vi "Main.vi"() -> ()   [LabVIEW 2017, in "My Singleton Module.lvlib"]
doc: "This template is based from the Queued Message Handler design pattern and the Queued Message Handler Project Template that ships with LabVIEW 2014.\n\nThe main difference is that the Queue is private to this module and communication between modules is done via Broadcast and Request events.\n\nRequest events are wrapped via public API methods and are handled in the Event handler loop in this VI.\nAny module can register for Broadcast events sent by this module.\n\nThe Event Handling Loop generates messages based on user interface actions.\n\nThe Message Handling Loop processes messages generated by the Event Handling Loop, or by other messages. The messages are string values, so new messages can be added easily to the Message Cases case structure in the Message Handling Loop. Each message cluster can also provide an optional value for Message Data, which is a variant that can be converted to whatever message-specific data is required.\n_____\nBased on Delacor QMH Project Template 3.1.0.34."
uses:
  My Singleton Module.lvlib
  <vilib>/Delacor/Delacor QMH/Libraries/Module Admin_class/Delacor_lib_QMH_Module Admin.lvclass
  Module Data--cluster.ctl
  Do Something Else Argument--cluster.ctl
  Do Something Else and Wait for Reply Argument--cluster.ctl
  Do Something Else and Wait (Reply Payload)--cluster.ctl
  Show Panel Argument--cluster.ctl
  Hide Panel Argument--cluster.ctl
  Stop Argument--cluster.ctl
  <vilib>/Delacor/Delacor QMH/Libraries/Module Admin_class/Delacor_lib_QMH_Module Admin.lvclass/Delacor_lib_QMH_Module Admin.ctl
  <vilib>/Utility/miscctls.llb/LVPointTypeDef.ctl
  <vilib>/Delacor/Delacor QMH/Libraries/Module Admin_class/Delacor_lib_QMH_Get External Launch.vi
  <vilib>/Delacor/Delacor QMH/Libraries/Message Queue_class/Delacor_lib_QMH_Enqueue Message (Single).vi
  <vilib>/Utility/error.llb/Error Cluster From Error Code.vi
  <vilib>/ErrorRing/Error Ring.xnode
  <vilib>/Delacor/Delacor QMH/Libraries/Message Queue_class/Delacor_lib_QMH_Message Queue.lvclass
panel:
  in  "Simulate MHL Error":bool
  in  "Simulate EHL Error":bool
  out "error out":errorcluster
  in  "Module Admin":refnum<class "Delacor_lib_QMH_Module Admin.lvclass">
  out "X":dbl
  out "Status":string
  in  "Do Something Else <Replace Me>":bool
  in  "Do Something <Replace Me>":bool
  # "These controls have associated \"Value Changed\" events configured in the Event Structure on the diagram.\n\nReplace them (and reconfigure the Event Structure) with the controls you need for your application. \n\nOther QMH Modules communicate with this Module via its Public API (wrappers for its Request Events).\n\nThis Module communicates with other Modules via its Broadcast Events.\nAny module that wants to get these messages, just registers for this module's Broadcast events."
  # "This template is for the Delacor Modified Queued Message Handler design pattern.\n\nSee the block diagram for more information on how to use this template."
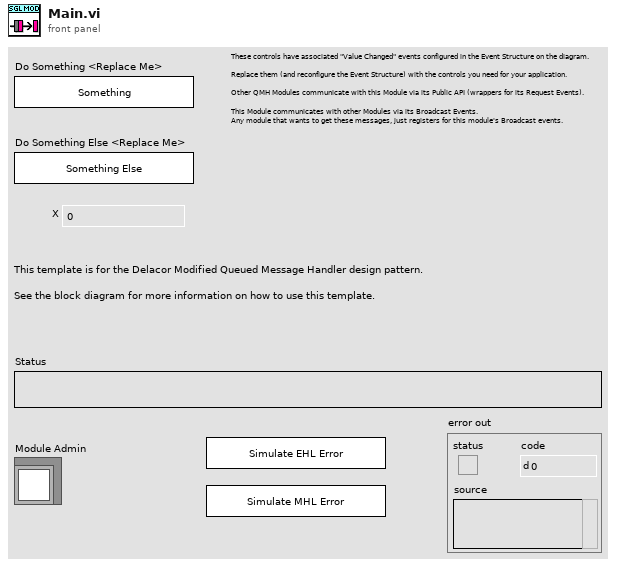
[diagram p1: front panel]
types:
  T1 = typedef "My Singleton Module.lvlib/Request Events--cluster.ctl" = cluster{"Stop Module":refnum<user-event>, "Do Something":refnum<user-event>, "Do Something Else":refnum<user-event>, "Do Something Else and Wait for Reply":refnum<user-event>, "Show Panel":refnum<user-event>, "Hide Panel":refnum<user-event>, "Get Module Execution Status":refnum<user-event>, "Show Diagram":refnum<user-event>}
  T2 = typedef "My Singleton Module.lvlib/Module Data--cluster.ctl" = cluster{"Status":string}
  T3 = typedef "My Singleton Module.lvlib/Do Something Else Argument--cluster.ctl" = cluster{"Do Something Else Msg":string, "X":dbl}
  T4 = typedef "My Singleton Module.lvlib/Do Something Else and Wait for Reply Argument--cluster.ctl" = cluster{"Do Something Else Msg":string, "X":dbl, "Wait Notifier":refnum<notifier>}
  T5 = typedef "My Singleton Module.lvlib/Show Panel Argument--cluster.ctl" = cluster{"Show Panel?":bool}
  T6 = typedef "My Singleton Module.lvlib/Hide Panel Argument--cluster.ctl" = cluster{"Hide Panel?":bool}
  T7 = typedef "My Singleton Module.lvlib/Stop Argument--cluster.ctl" = cluster{"Origin":string, "Exit via Stop Module Req?":bool, "Wait for Module to stop?":bool}
  T8 = typedef "LVPointTypeDef.ctl" = cluster{"Horizontal":i16, "Vertical":i16}
  T9 = enum32{"Invalid", "Standard", "Closed", "Hidden", "Minimized", "Maximized"}
  T10 = enum32{"invalid lock state", "Not Locked", "Locked (No Password)", "Password-protected"}
  T11 = typedef "My Singleton Module.lvlib/Do Something Else and Wait (Reply Payload)--cluster.ctl" = cluster{"Value":dbl, "error":errorcluster}
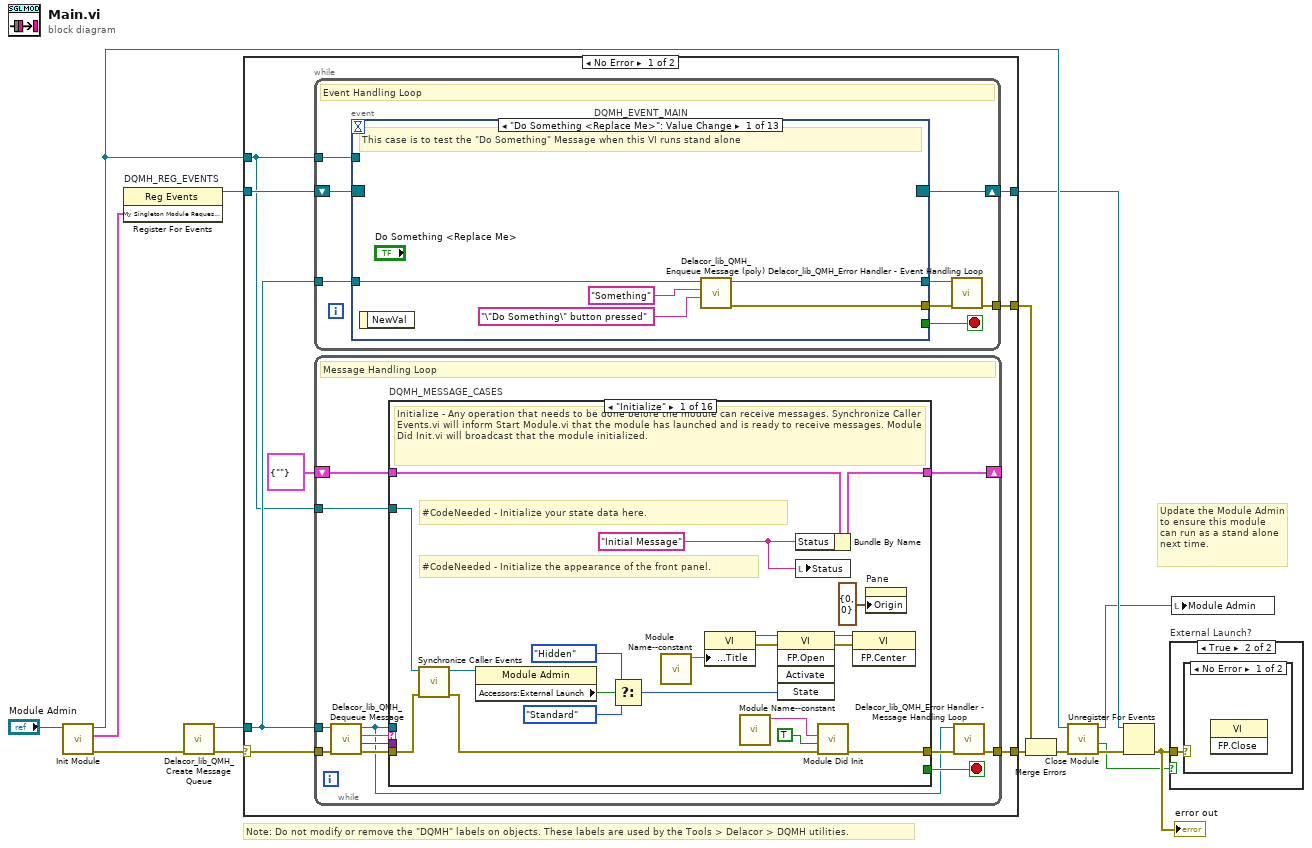
[diagram p0: block diagram]
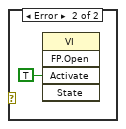
[diagram p3: hidden frame]
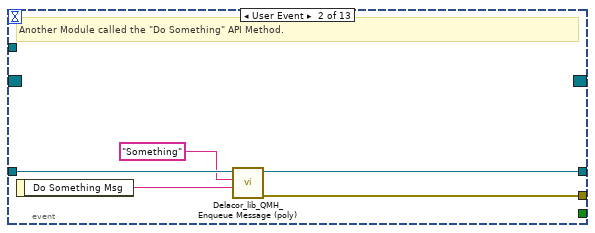
[diagram p4: hidden frame]
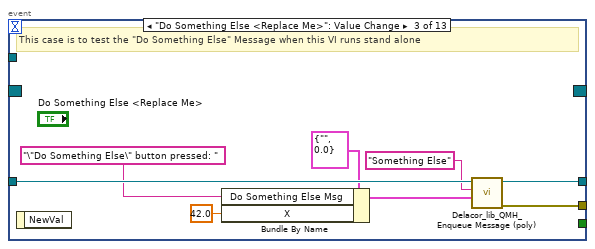
[diagram p5: hidden frame]
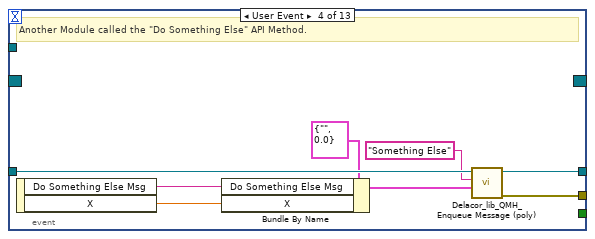
[diagram p6: hidden frame]
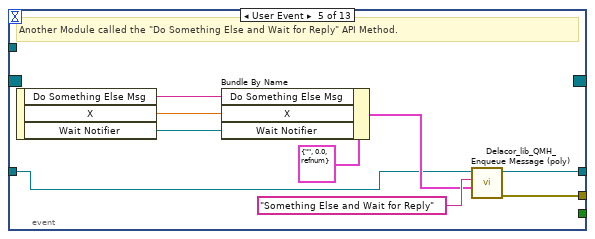
[diagram p7: hidden frame]
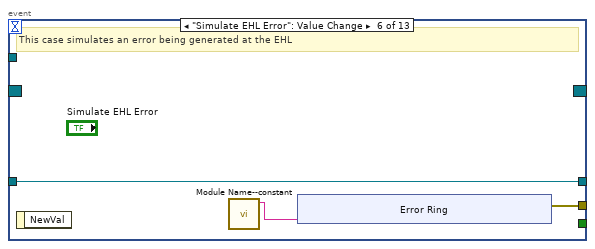
[diagram p8: hidden frame]
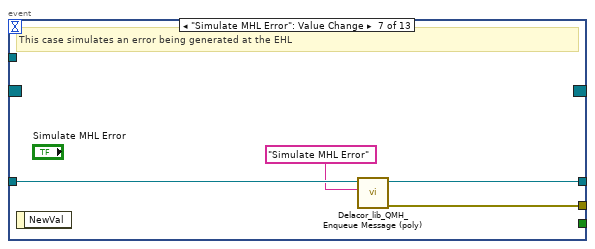
[diagram p9: hidden frame]
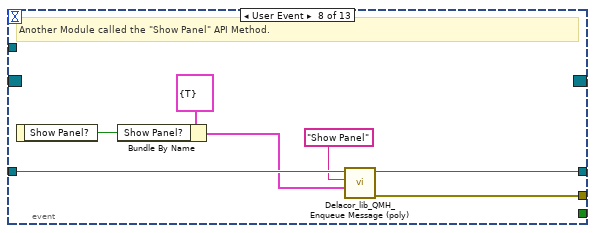
[diagram p10: hidden frame]
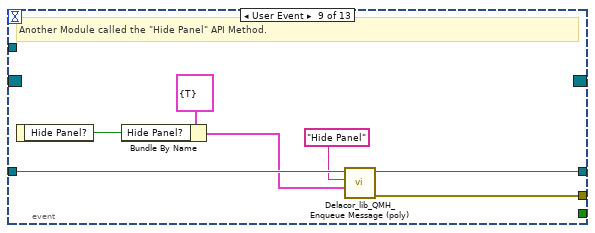
[diagram p11: hidden frame]
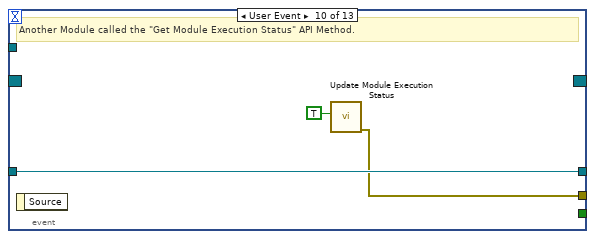
[diagram p12: hidden frame]
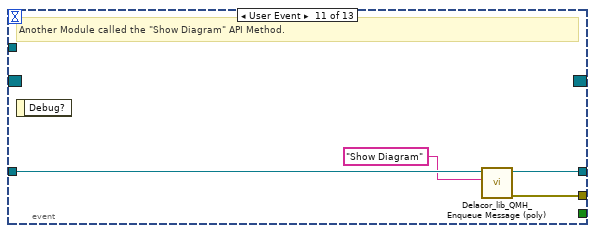
[diagram p13: hidden frame]
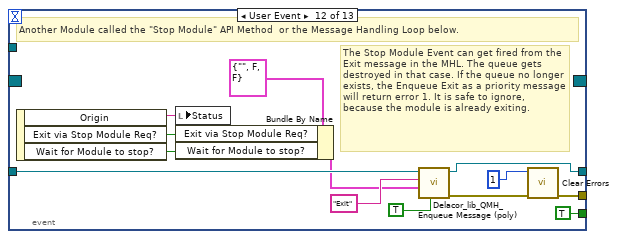
[diagram p14: hidden frame]
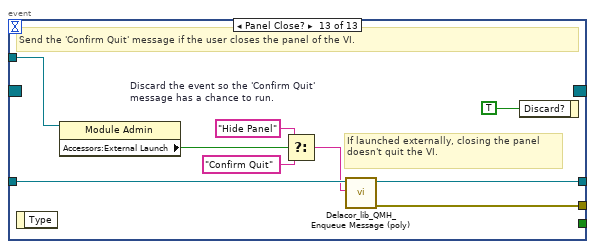
[diagram p15: hidden frame]
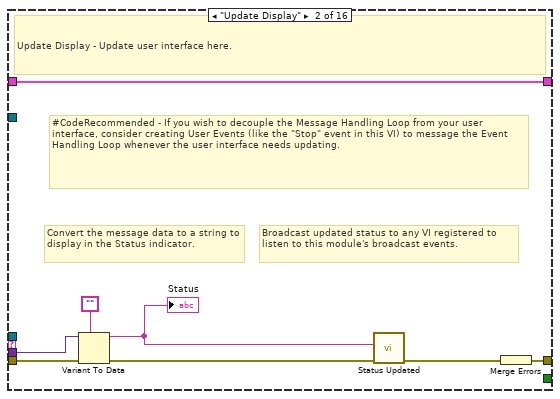
[diagram p16: hidden frame]
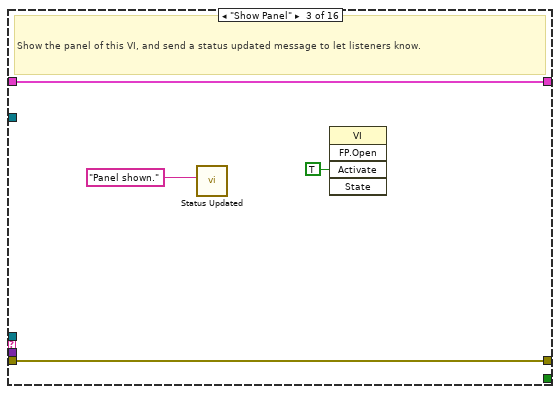
[diagram p17: hidden frame]
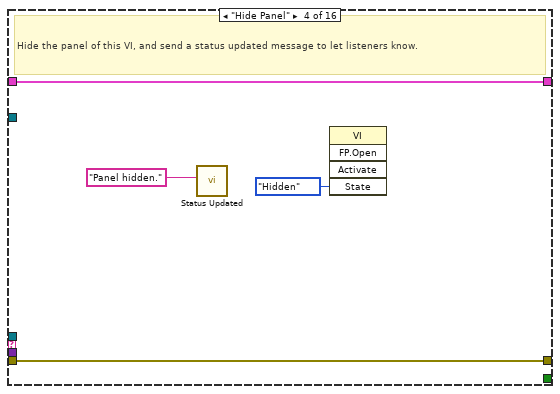
[diagram p18: hidden frame]
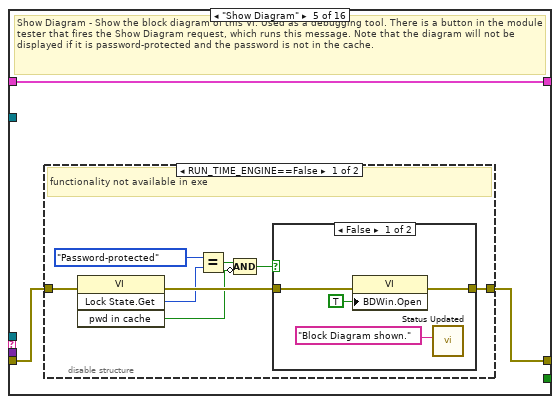
[diagram p19: hidden frame]
diagram:
  # "Note: Do not modify or remove the \"DQMH\" labels on objects. These labels are used by the Tools > Delacor > DQMH utilities."
  # "Update the Module Admin to ensure this module can run as a stand alone next time."
  n1 = call "Init Module.vi"("Singleton Module Admin in"="Module Admin") -> ("error out"=w13:errorcluster, "My Singleton Module Request Events"=w10:T1, "Singleton Module Admin out"=w15:refnum<class "Delacor_lib_QMH_Module Admin.lvclass">)  [unwired: 8 in]
  n2 = register-events "DQMH_REG_EVENTS"(w10) -> (reference out=w11:refnum<event-registration>)  [unwired: 2 in, 1 out]
  n3 = call <vilib>:"Delacor_lib_QMH_Create Message Queue.vi"("error in (no error)"=w13) -> ("error out"=w1:errorcluster, "Message Queue out"=w9:refnum<class "Delacor_lib_QMH_Message Queue.lvclass">)  [unwired: 9 in]
  n4 = case shown="No Error" w1 {
    selector: w1 -> [w17 w316]
    tunnel: [w23 w316] -> w14
    tunnel: [w22 w321] -> w12
    tunnel: w11 -> [w20 w321]
    tunnel: w9 -> [w19 _]
    tunnel: [w18 _] -> w5
    tunnel: w15 -> [w16 w317]
    frame No Error {
      n5 = while {
        tunnel: w19 -> [w31]
        shift-right: [w29] -> w22
        shift-left: w20 -> [w30]
        tunnel: [w25] -> w18
        tunnel: w16 -> [w24]
        stop <- w27 stop-if-true
        # "Event Handling Loop"
        n6 = event "DQMH_EVENT_MAIN" shown="[0] \"Do Something <Replace Me>\": Value Change" {
          selector: w30 -> [_ _ _ _ _ _ _ _ _ _ _ _ _]
          dyn-events: [_ _ _ _ _ _ _ _ _ _ _ _ _] -> w29
          timeout: _ -> [_ _ _ _ _ _ _ _ _ _ _ _ _]
          tunnel: [_ _ _ _ _ _ _ _ _ _ _ TRUE ("Discard?") _] -> w27
          tunnel: w31 -> [w36 w41 w49 w57 w58 w69 w80 w87 w94 w97 w101 w112 w122]
          tunnel: [w33 w38 w46 w54 w64 w68 w77 w85 w92 w96 w98 w106 w121] -> w28
          tunnel: [w35 w40 w48 w56 w66 w69 w79 w86 w93 w97 w100 w111 w120] -> w26
          tunnel: w24 -> [_ _ _ _ _ _ _ _ _ _ _ _ w116]
          event "Do Something <Replace Me>": Value Change {
            # "This case is to test the \"Do Something\" Message when this VI runs stand alone"
            n7 = event-data() -> ()  [unwired: 1 in, 1 out]
            n8 = call-poly <vilib>:"Delacor_lib_QMH_Enqueue Message (poly).vi"("Message Data"="\"Do Something\" button pressed" ("\"Do Something\" button pressed"), "Message"="Something", "Message Queue in"=w36) -> ("error out"=w33:errorcluster, "Message Queue out"=w35:refnum<class "Delacor_lib_QMH_Message Queue.lvclass">)  [unwired: 7 in]
          }
          event User Event {
            # "Another Module called the \"Do Something\" API Method."
            n9 = event-data() -> ("Do Something Msg"=w37:string)  [unwired: 1 in]
            n10 = call-poly <vilib>:"Delacor_lib_QMH_Enqueue Message (poly).vi"("Message Data"=w37, "Message"="Something", "Message Queue in"=w41) -> ("error out"=w38:errorcluster, "Message Queue out"=w40:refnum<class "Delacor_lib_QMH_Message Queue.lvclass">)  [unwired: 7 in]
          }
          event "Do Something Else <Replace Me>": Value Change {
            # "This case is to test the \"Do Something Else\" Message when this VI runs stand alone"
            n11 = event-data() -> ()  [unwired: 1 in, 1 out]
            n12 = Bundle By Name(cluster=T3 {"Do Something Else Msg"="", "X"=0.0} ("Do Something Else Argument"), "Do Something Else Msg"="\"Do Something Else\" button pressed: " ("\"Do Something Else\" button pressed"), "X"=42.0) -> (w44:T3)
            n13 = call-poly <vilib>:"Delacor_lib_QMH_Enqueue Message (poly).vi"("Message Data"=w44, "Message"="Something Else", "Message Queue in"=w49) -> ("error out"=w46:errorcluster, "Message Queue out"=w48:refnum<class "Delacor_lib_QMH_Message Queue.lvclass">)  [unwired: 7 in]
          }
          event User Event {
            # "Another Module called the \"Do Something Else\" API Method."
            n14 = event-data() -> ("Do Something Else Msg"=w51:string, "X"=w50:dbl)  [unwired: 1 in]
            n15 = Bundle By Name(cluster=T3 {"Do Something Else Msg"="", "X"=0.0} ("Do Something Else Argument"), "Do Something Else Msg"=w51, "X"=w50) -> (w52:T3)
            n16 = call-poly <vilib>:"Delacor_lib_QMH_Enqueue Message (poly).vi"("Message Data"=w52, "Message"="Something Else", "Message Queue in"=w57) -> ("error out"=w54:errorcluster, "Message Queue out"=w56:refnum<class "Delacor_lib_QMH_Message Queue.lvclass">)  [unwired: 7 in]
          }
          event User Event {
            # "Another Module called the \"Do Something Else and Wait for Reply\" API Method."
            n17 = event-data() -> ("Do Something Else Msg"=w61:string, "X"=w60:dbl, "Wait Notifier"=w59:refnum<notifier>)  [unwired: 1 in]
            n18 = Bundle By Name(cluster=T4 {"Do Something Else Msg"="", "X"=0.0, "Wait Notifier"=refnum} ("Do Something Else and Wait for Reply Argument"), "Do Something Else Msg"=w61, "X"=w60, "Wait Notifier"=w59) -> (w62:T4)
            n19 = call-poly <vilib>:"Delacor_lib_QMH_Enqueue Message (poly).vi"("Message Data"=w62, "Message"="Something Else and Wait for Reply", "Message Queue in"=w58) -> ("error out"=w64:errorcluster, "Message Queue out"=w66:refnum<class "Delacor_lib_QMH_Message Queue.lvclass">)  [unwired: 7 in]
          }
          event "Simulate EHL Error": Value Change {
            # "This case simulates an error being generated at the EHL"
            n20 = event-data() -> ()  [unwired: 1 in, 1 out]
            n21 = call "Module Name--constant.vi"() -> ("Module Name"=w67:string)  [unwired: 11 in]
            n22 = xnode "Error Ring"("parameter 0"=w67) -> ("error out"=w68:errorcluster)
          }
          event "Simulate MHL Error": Value Change {
            # "This case simulates an error being generated at the EHL"
            n23 = event-data() -> ()  [unwired: 1 in, 1 out]
            n24 = call-poly <vilib>:"Delacor_lib_QMH_Enqueue Message (poly).vi"("Message"="Simulate MHL Error", "Message Queue in"=w80) -> ("error out"=w77:errorcluster, "Message Queue out"=w79:refnum<class "Delacor_lib_QMH_Message Queue.lvclass">)  [unwired: 8 in]
          }
          event User Event {
            # "Another Module called the \"Show Panel\" API Method."
            n25 = event-data() -> ("Show Panel?"=w83:bool)  [unwired: 1 in]
            n26 = Bundle By Name(cluster=T5 {"Show Panel?"=TRUE} ("Show Panel Argument"), "Show Panel?"=w83) -> (w81:T5)
            n27 = call-poly <vilib>:"Delacor_lib_QMH_Enqueue Message (poly).vi"("Message Data"=w81, "Message"="Show Panel", "Message Queue in"=w87) -> ("error out"=w85:errorcluster, "Message Queue out"=w86:refnum<class "Delacor_lib_QMH_Message Queue.lvclass">)  [unwired: 7 in]
          }
          event User Event {
            # "Another Module called the \"Hide Panel\" API Method."
            n28 = event-data() -> ("Hide Panel?"=w89:bool)  [unwired: 1 in]
            n29 = Bundle By Name(cluster=T6 {"Hide Panel?"=TRUE} ("Hide Panel Argument"), "Hide Panel?"=w89) -> (w88:T6)
            n30 = call-poly <vilib>:"Delacor_lib_QMH_Enqueue Message (poly).vi"("Message Data"=w88, "Message"="Hide Panel", "Message Queue in"=w94) -> ("error out"=w92:errorcluster, "Message Queue out"=w93:refnum<class "Delacor_lib_QMH_Message Queue.lvclass">)  [unwired: 7 in]
          }
          event User Event {
            # "Another Module called the \"Get Module Execution Status\" API Method."
            n31 = event-data() -> ()  [unwired: 1 in, 1 out]
            n32 = call "Update Module Execution Status.vi"("Running?"=TRUE) -> ("error out"=w96:errorcluster)  [unwired: 10 in]
          }
          event User Event {
            # "Another Module called the \"Show Diagram\" API Method."
            n33 = event-data() -> ()  [unwired: 1 in, 1 out]
            n34 = call-poly <vilib>:"Delacor_lib_QMH_Enqueue Message (poly).vi"("Message"="Show Diagram", "Message Queue in"=w101) -> ("error out"=w98:errorcluster, "Message Queue out"=w100:refnum<class "Delacor_lib_QMH_Message Queue.lvclass">)  [unwired: 8 in]
          }
          event User Event {
            # "The Stop Module Event can get fired from the Exit message in the MHL. The queue gets destroyed in that case. If the queue no longer exists, the Enqueue Exit as a priority message will return error 1. It is safe to ignore, because the module is already exiting."
            # "Another Module called the \"Stop Module\" API Method  or the Message Handling Loop below."
            n35 = event-data() -> ("Origin"=w110:string, "Exit via Stop Module Req?"=w104:bool, "Wait for Module to stop?"=w103:bool)  [unwired: 1 in]
            n36 = local write "Status"(w110) -> ()
            n37 = Bundle By Name(cluster=T7 {"Origin"="", "Exit via Stop Module Req?"=FALSE, "Wait for Module to stop?"=FALSE} ("Stop Argument"), "Exit via Stop Module Req?"=w104, "Wait for Module to stop?"=w103) -> (w102:T7)
            n38 = call-poly <vilib>:"Delacor_lib_QMH_Enqueue Message (poly).vi"("Priority Message? (F)"=TRUE, "Message Data"=w102, "Message"="Exit", "Message Queue in"=w112) -> ("error out"=w107:errorcluster, "Message Queue out"=w111:refnum<class "Delacor_lib_QMH_Message Queue.lvclass">)  [unwired: 6 in]
            n39 = call <vilib>:"Clear Errors.vi"("error in (no error)"=w107, "specific error code to clear (0: all)"=1) -> ("error out"=w106:errorcluster)  [unwired: 4 in, 1 out]
          }
          event Panel Close? {
            w123 = TRUE  # Discard the event so the 'Confirm Quit' message has a chance to run.
            # "If launched externally, closing the panel doesn't quit the VI."
            # "Send the 'Confirm Quit' message if the user closes the panel of the VI."
            n40 = event-data() -> ()  [unwired: 1 in, 1 out]
            n41 = property class="Module Admin"(reference=w116) -> ("Accessors:External Launch"=w115:bool)  [unwired: 1 in, 2 out]
            n42 = Select(t="Hide Panel" ("Message"), s=w115, f="Confirm Quit" ("Message")) -> (s? t:f=w117:string)
            n43 = call-poly <vilib>:"Delacor_lib_QMH_Enqueue Message (poly).vi"("Message"=w117, "Message Queue in"=w122) -> ("error out"=w121:errorcluster, "Message Queue out"=w120:refnum<class "Delacor_lib_QMH_Message Queue.lvclass">)  [unwired: 8 in]
            n44 = event-data("Discard?"=w123) -> ()  [unwired: 1 in, 1 out]
          }
        }
        n45 = call-dynamic "Delacor_lib_QMH_Error Handler - Event Handling Loop.vi"("error in (no error)"=w28, "Message Queue in"=w26) -> ("dup error in"=w25:errorcluster)  [unwired: 8 in, 1 out]
      }
      n46 = while {
        tunnel: w19 -> [w127]
        shift-right: [w133] -> _
        shift-left: T2 {"Status"=""} ("Data Cluster") -> [w134]
        tunnel: w17 -> [w131]
        tunnel: [w125] -> w23
        tunnel: w16 -> [w124]
        stop <- w132 stop-if-true
        # "Message Handling Loop"
        n47 = call-dynamic "Delacor_lib_QMH_Dequeue Message.vi"("error in (no error)"=w131, "Message Queue in"=w127) -> ("error out"=w130:errorcluster, "Message Data"=w128:variant, "Message"=w129:string, "Message Queue out"=w126:refnum<class "Delacor_lib_QMH_Message Queue.lvclass">)  [unwired: 6 in]
        n48 = case "DQMH_MESSAGE_CASES" shown="\"Initialize\"" w129 {
          selector: w129 -> [_ _ _ _ _ _ _ _ _ _ _ _ _ _ _ w303]
          tunnel: w126 -> [_ _ _ _ _ _ w197 w212 w235 _ _ _ w267 w282 w299 _]
          tunnel: w130 -> [w145 w161 w167 w168 w173 w191 w202 w210 w233 w248 w251 w256 w273 w286 w301 _]
          tunnel: [w138 w162 w167 w168 w172 w189 w199 w214 w217 w246 w249 w254 w264 w284 w295 w304] -> w135
          tunnel: w134 -> [w144 w163 w166 w171 w174 w190 w200 w215 w237 w247 w250 w255 w272 w285 w298 w305]
          tunnel: [w143 w163 w166 w171 w174 w190 w200 w215 w237 w247 w250 w255 w272 w285 w298 w305] -> w133
          tunnel: [_ _ _ _ _ _ _ _ _ _ _ _ _ _ w297 _] -> w132
          tunnel: w128 -> [_ w160 _ _ _ _ w194 w206 w229 _ _ _ w271 _ w294 _]
          tunnel: w124 -> [w146 _ _ _ _ _ _ _ _ _ _ _ w266 _ w287 _]
          frame "Initialize" {
            w142 = "Initial Message" ("Initial Message")
            # "#CodeNeeded - Initialize the appearance of the front panel."
            # "#CodeNeeded - Initialize your state data here."
            # "Initialize - Any operation that needs to be done before the module can receive messages. Synchronize Caller Events.vi will inform Start Module.vi that the module has launched and is ready to receive messages. Module Did Init.vi will broadcast that the module initialized."
            n49 = call "Synchronize Caller Events.vi"("error in (no error)"=w145, "Singleton Module Admin in"=w146) -> ("error out"=w139:errorcluster, "Singleton Module Admin out"=w137:refnum<class "Delacor_lib_QMH_Module Admin.lvclass">)  [unwired: 8 in]
            n50 = property class="Module Admin"(reference=w137) -> ("Accessors:External Launch"=w150:bool)  [unwired: 1 in, 2 out]
            n51 = Select(t=T9."Hidden" ("State"), s=w150, f=T9."Standard" ("State")) -> (s? t:f=w147:T9)
            n52 = call "Module Name--constant.vi"() -> ("Module Name"=w155:string)  [unwired: 11 in]
            n53 = property class="VI"("Front Panel.Title"=w155) -> (reference out=w153:refnum<vi>, error out=w154:errorcluster)  [unwired: 2 in]
            n54 = call "Module Name--constant.vi"() -> ("Module Name"=w140:string)  [unwired: 11 in]
            n55 = invoke class="VI" method="FP.Open"(reference=w153, error in=w154, "State"=w147) -> (reference out=w152:refnum<vi>, error out=w151:errorcluster)  [unwired: 2 in, 3 out]
            n56 = Bundle By Name(cluster=w144, "Status"=w142) -> (w143:T2)
            n57 = local write "Status"(w142) -> ()
            n58 = call "Module Did Init.vi"("error in (no error)"=w139, "Initialized?"=TRUE, "Origin"=w140) -> ("error out"=w138:errorcluster)  [unwired: 8 in]
            n59 = invoke class="VI" method="FP.Center"(reference=w152, error in=w151) -> ()  [unwired: 1 in, 3 out]
            n60 = property on="Pane" class="Pane"("Origin"=T8 {"Horizontal"=0, "Vertical"=0}) -> ()  [unwired: 2 in, 2 out]
          }
          frame "Update Display" {
            # "Broadcast updated status to any VI registered to listen to this module's broadcast events."
            # "Convert the message data to a string to display in the Status indicator."
            # "#CodeRecommended - If you wish to decouple the Message Handling Loop from your user interface, consider creating User Events (like the \"Stop\" event in this VI) to message the Event Handling Loop whenever the user interface needs updating."
            # "Update Display - Update user interface here."
            n61 = Variant To Data(error in=w161, type="", Variant=w160) -> (data=w158:string, error out=w157:errorcluster)
            "Status" <- w158
            n62 = call "Status Updated.vi"("error in (no error)"=w157, "Status"=w158) -> ("error out"=w156:errorcluster)  [unwired: 9 in]
            n63 = Merge Errors(w156) -> (w162:errorcluster)
          }
          frame "Show Panel" {
            # "Show the panel of this VI, and send a status updated message to let listeners know."
            n64 = call "Status Updated.vi"("Status"="Panel shown." ("format string")) -> ()  [unwired: 10 in, 1 out]
            n65 = invoke class="VI" method="FP.Open"("Activate"=TRUE ("Activate?")) -> ()  [unwired: 4 in, 5 out]
          }
          frame "Hide Panel" {
            # "Hide the panel of this VI, and send a status updated message to let listeners know."
            n66 = call "Status Updated.vi"("Status"="Panel hidden." ("format string")) -> ()  [unwired: 10 in, 1 out]
            n67 = invoke class="VI" method="FP.Open"("State"=T9."Hidden") -> ()  [unwired: 4 in, 5 out]
          }
          frame "Show Diagram" {
            # "Show Diagram - Show the block diagram of this VI. Used as a debugging tool. There is a button in the module tester that fires the Show Diagram request, which runs this message. Note that the diagram will not be displayed if it is password-protected and the password is not in the cache."
            n68 = disable-structure shown="RUN_TIME_ENGINE==False" {
              disable-tunnel: [w182 w188] -> w172
              disable-tunnel: w173 -> [w181 w188]
              frame condition #0 (active) {
                # "functionality not available in exe"
                n69 = invoke class="VI" method="Lock State.Get"(error in=w181) -> (error out=w180:errorcluster, "Get Lock State"=w179:T10, "pwd in cache"=w176:bool)  [unwired: 3 in, 1 out]
                n70 = Equal?(x=T10."Password-protected", y=w179) -> (x = y?=w177:bool)
                n71 = Compound Arithmetic op=AND(w177, invert w176) -> (w175:bool)
                n72 = case shown="False" w175 {
                  tunnel: [w185 w187] -> w182
                  tunnel: w180 -> [w183 w187]
                  frame False {
                    n73 = property class="VI"(error in=w183, "BDWin.Open"=TRUE ("Block Diagram Window:Open")) -> (error out=w185:errorcluster)  [unwired: 1 in, 1 out]
                    n74 = call "Status Updated.vi"("Status"="Block Diagram shown." ("format string")) -> ()  [unwired: 10 in, 1 out]
                  }
                  frame True {
                    # "Password-protected VI, and the password is not in the cache. Do not show the diagram."
                  }
                }
              }
              frame condition #1 {
              }
            }
          }
          frame "--- Module Specific ---" {
            # "Separator -- The following cases handle messages specific to this Module."
            n75 = Merge Errors(w191) -> (w189:errorcluster)
          }
          frame "Something" {
            # "Send string to \"Update Display\" message"
            # "#CodeNeeded - Perform whatever actions correspond to the \"Something\" message."
            # "Something - Replace this message with functionality for your own application. Note that this message also fires the round-trip \"Did Something\" broadcast event."
            n76 = Variant To Data(error in=w202, type="", Variant=w194) -> (data=w192:string, error out=w201:errorcluster)
            n77 = call "Did Something.vi"("error in (no error)"=w201, "Did Something Msg"=w192) -> ("error out"=w193:errorcluster)  [unwired: 9 in]
            n78 = call-poly <vilib>:"Delacor_lib_QMH_Enqueue Message (poly).vi"("error in (no error)"=w201, "Message Data"=w192, "Message"="Update Display", "Message Queue in"=w197) -> ("error out"=w198:errorcluster)  [unwired: 6 in, 1 out]
            n79 = Merge Errors(w193, w198) -> (w199:errorcluster)
          }
          frame "Something Else" {
            # "Send string to \"Update Display\" message"
            # "#CodeNeeded - Perform whatever actions correspond to the \"Something Else\" message."
            # "Something Else - Replace this message with functionality for your own application."
            n80 = Variant To Data(error in=w210, type=T3 {"Do Something Else Msg"="", "X"=0.0} ("Do Something Else Argument"), Variant=w206) -> (data=w207:T3, error out=w209:errorcluster)
            n81 = Unbundle By Name(w207) -> ("Do Something Else Msg"=w205:string, "X"=w203:dbl)
            "X" <- w203
            n82 = Format Into String(initial string=w205, w203) -> (resulting string=w204:string)  [unwired: 2 in, 1 out]
            n83 = call-poly <vilib>:"Delacor_lib_QMH_Enqueue Message (poly).vi"("error in (no error)"=w209, "Message Data"=w204, "Message"="Update Display", "Message Queue in"=w212) -> ("error out"=w213:errorcluster)  [unwired: 6 in, 1 out]
            n84 = Merge Errors(w213) -> (w214:errorcluster)
          }
          frame "Something Else and Wait for Reply" {
            w220 = "X(%.2f)+Offset(%.2f)=%.2f"  # status message format string
            # "Send back X with a random offset"
            # "Something Else and Wait for Reply - Replace this message with functionality for your own application. Note that this message must fire a notifier to let callers know it has finished execution, and it returns an error if the 'Value' is negative."
            n85 = Random Number (0-1)() -> (number: 0 to 1=w222:dbl)
            n86 = Variant To Data(error in=w233, type=T4 {"Do Something Else Msg"="", "X"=0.0, "Wait Notifier"=refnum} ("Do Something Else and Wait for Reply Argument"), Variant=w229) -> (data=w230:T4, error out=w232:errorcluster)
            n87 = Unbundle By Name(w230) -> ("Wait Notifier"=w226:refnum<notifier>, "Do Something Else Msg"=w228:string, "X"=w221:dbl)
            n88 = Add(x=w222, y=w221) -> (x+y=w219:dbl)
            n89 = local write "X"(w221) -> ()
            n90 = flat-sequence {
              tunnel: w226 -> [w245]
              tunnel: [w245] -> w225
              frame #0 {
                # "Simulate an operation that requires a wait."
                n91 = Wait (ms)(milliseconds to wait=u32 1000) -> ()  [unwired: 1 out]
              }
            }
            n92 = Less Than 0?(x=w219) -> (x < 0?=w218:bool)
            n93 = case shown="True" w218 {
              tunnel: [_ w238] -> w216
              frame False {
              }
              frame True {
                n94 = xnode "Error Ring"() -> ("error out"=w238:errorcluster)
              }
            }
            n95 = Format Into String(format string=w220, initial string=w228, w221, w222, w219) -> (resulting string=w227:string)  [unwired: 1 in, 1 out]
            n96 = Bundle By Name(cluster=T11 {"Value"=0.0, "error"={"status"=FALSE, "code"=0, "source"=""}} ("notification"), "Value"=w219, "error"=w216) -> (w223:T11)
            n97 = call-poly <vilib>:"Delacor_lib_QMH_Enqueue Message (poly).vi"("error in (no error)"=w232, "Message Data"=w227, "Message"="Update Display", "Message Queue in"=w235) -> ("error out"=w236:errorcluster)  [unwired: 6 in, 1 out]
            n98 = Send Notification(notification=w223, notifier=w225) -> ()  [unwired: 1 in, 2 out]
            n99 = Merge Errors(w216, w236) -> (w217:errorcluster)
          }
          frame "---Copy This Frame---" {
            # "Duplicate this frame when creating new messages.  Change this comment in the duplicated frame to describe this message."
            n100 = Merge Errors(w248) -> (w246:errorcluster)
          }
          frame "--- Exit and Error Handling---" {
            # "Separator - The following cases handle errors and exit messages."
            n101 = Merge Errors(w251) -> (w249:errorcluster)
          }
          frame "Simulate MHL Error" {
            # "Simulate an error occurring at the MHL"
            n102 = call "Module Name--constant.vi"() -> ("Module Name"=w253:string)  [unwired: 11 in]
            n103 = xnode "Error Ring"("parameter 0"=w253) -> ("error out"=w252:errorcluster)
            n104 = Merge Errors(w256, w252) -> (w254:errorcluster)
          }
          frame "Error" {
            # "#CodeRecommended - If you ever change the name of this \"Error\" message, you'll need to update the name in the Check Loop Error.vi as well."
            # "#CodeRecommended - If the module is running in standalone mode (External Launch = FALSE), this code will pop up an error dialog and call the 'Exit' message if an error occurs. Add more fine-grained error handling here."
            # "Error - Check the error message data and respond accordingly. This message is sent by the \"Error Handler\" VIs at the end of each loop in this application."
            n105 = property class="Module Admin"(reference=w266) -> ("Accessors:External Launch"=w265:bool)  [unwired: 1 in, 2 out]
            n106 = Variant To Data(error in=w273, type=errorcluster {"status"=FALSE, "code"=0, "source"=""} ("error constant"), Variant=w271) -> (data=w274:errorcluster, error out=w269:errorcluster)
            n107 = call "Error Reported.vi"("Error"=w274) -> ()  [unwired: 10 in, 1 out]
            n108 = case shown="False" w265 {
              tunnel: [w279 _] -> w268
              tunnel: w267 -> [w278 _]
              tunnel: w274 -> [w275 _]
              frame False {
                # "If the module is running standalone, then pop up an error dialog and call the \"Exit\" message."
                n109 = call <vilib>:"Simple Error Handler.vi"("error in (no error)"=w275) -> ()  [unwired: 4 in, 5 out]
                n110 = call-poly <vilib>:"Delacor_lib_QMH_Enqueue Message (poly).vi"("Priority Message? (F)"=TRUE, "Message"="Exit", "Message Queue in"=w278) -> ("error out"=w279:errorcluster)  [unwired: 7 in, 1 out]
              }
              frame True {
                # "If the module was launched externally, calling the Error Reported broadcast VI is the only action performed by the \"Error\" message. The module's caller can then process the error appropriately."
              }
            }
            n111 = Merge Errors(w269, w268) -> (w264:errorcluster)
            n112 = local write "error out"(w264) -> ()
          }
          frame "Confirm Quit" {
            # "#CodeNeeded - If you want to provide an \"Are you sure\" dialog (or some other notification) before the application exits, place that code here. This message is typically sent from a Panel Close? event."
            # "Confirm Quit - Message that can confirm whether or not the user wants to exit the application."
            n113 = call-poly <vilib>:"Delacor_lib_QMH_Enqueue Message (poly).vi"("Priority Message? (F)"=TRUE, "error in (no error)"=w286, "Message"="Exit", "Message Queue in"=w282) -> ("error out"=w283:errorcluster)  [unwired: 6 in, 1 out]
            n114 = Merge Errors(w283) -> (w284:errorcluster)
          }
          frame "Exit" {
            w292 = 91  # 91: not all Exit messages will have an argument
            w297 = TRUE  # Stop the VI
            # "Release the message queue reference"
            # "#CodeNeeded - Add any required cleanup code here"
            # "Exit - Exit the application."
            n115 = Variant To Data(error in=w301, type=T7 {"Origin"="", "Exit via Stop Module Req?"=FALSE, "Wait for Module to stop?"=FALSE} ("Stop Argument"), Variant=w294) -> (data=w290:T7, error out=w293:errorcluster)
            n116 = call <vilib>:"Clear Errors.vi"("error in (no error)"=w293, "specific error code to clear (0: all)"=w292) -> ("error out"=w300:errorcluster)  [unwired: 4 in, 1 out]
            n117 = control-ref of="This VI"() -> (w288:refnum<vi>)
            n118 = call-dynamic "Delacor_lib_QMH_Release Message Queue.vi"("error in (no error)"=w300, "Message Queue"=w299) -> ("error out"=w296:errorcluster)  [unwired: 9 in]
            n119 = call "Handle Exit.vi"("Stop Argument"=w290, "Admin in"=w287, "VI reference"=w288) -> ("error out"=w289:errorcluster)  [unwired: 7 in, 1 out]
            n120 = Merge Errors(w289, w296) -> (w295:errorcluster)
          }
          frame Default {
            # "'Default' case only runs if there is a message that isn't defined in any of the other cases.  Output a programming error."
            n121 = call "Module Name--constant.vi"() -> ("Module Name"=w302:string)  [unwired: 11 in]
            n122 = xnode "Error Ring"("parameter 0"=w303, "parameter 1"=w302) -> ("error out"=w304:errorcluster)
          }
        }
        n123 = call-dynamic "Delacor_lib_QMH_Error Handler - Message Handling Loop.vi"("error in (no error)"=w135, "Message Queue in"=w126) -> ("dup error in"=w125:errorcluster)  [unwired: 8 in, 1 out]
      }
    }
    frame Error {
      # "Synchronize Caller Events.vi will inform Start Module.vi that the module has launched and will let the code calling Start Module.vi register for broadcasts and would permit the caller receive the broadcast that an error occurred at launch time."
      n124 = call "Synchronize Caller Events.vi"("Singleton Module Admin in"=w317) -> ("error out"=w314:errorcluster)  [unwired: 9 in, 1 out]
      n125 = call "Module Name--constant.vi"() -> ("Module Name"=w320:string)  [unwired: 11 in]
      n126 = Format Into String(format string="An error occurred during initialization. %s is no longer running.", w320) -> (resulting string=w318:string)  [unwired: 2 in, 1 out]
      n127 = Merge Errors(w316, w314) -> (w315:errorcluster)
      n128 = call "Error Reported.vi"("Additional Information"=w318, "Error"=w315) -> ()  [unwired: 9 in, 1 out]
    }
  }
  n129 = Merge Errors(w5, w14) -> (w4:errorcluster)
  n130 = call "Close Module.vi"("error in (no error)"=w4, "Module Admin in"=w15) -> ("error out"=w7:errorcluster, "External Launch"=w2:bool, "Module Admin out"=w6:refnum<class "Delacor_lib_QMH_Module Admin.lvclass">)  [unwired: 7 in]
  n131 = Unregister For Events(event registration refnum=w12, error in=w7) -> (error out=w3:errorcluster)
  "error out" <- w3
  n132 = case "External Launch?" shown="True" w2 {
    tunnel: w3 -> [_ w322]
    frame False {
    }
    frame True {
      n133 = case shown="No Error" w322 {
        frame No Error {
          n134 = invoke class="VI" method="FP.Close"() -> ()  [unwired: 3 in, 3 out]
        }
        frame Error {
          n135 = invoke class="VI" method="FP.Open"("Activate"=TRUE ("Activate?")) -> ()  [unwired: 4 in, 5 out]
        }
      }
    }
  }
  n136 = local write "Module Admin"(w6) -> ()
